vi "GUI_kHz_AlpaoWFS.vi"() -> ()   [LabVIEW 2020]
uses:
  Shared/GUI_Template/GUI_master/tcp_new_data_event.ctl
  Shared/GUI_Template/GUI_master/tcp new data cluster.ctl
  <vilib>/vision/Image Controls.llb/IMAQ Image.ctl
  <vilib>/vision/NI_Vision_Development_Module.lvlib
panel:
  in  "save::1":bool caption="Save"
  in  "exposure::1":dbl=1.005311 caption="Exposure" min=0.001 max=10000.0 format="%_3p"
  in  "cameraselect::1":enum16{"temporal CAM", "spatial CAM"}(ring) caption="Select Camera"
  in  "triggermode::1":bool=TRUE caption="Blank Button"
  in  "Select device":string(combo)="kHz_WFS_Alpao"
  out "tcp data event 2":T1
  out "Tank":dbl(slide)=42.0 scale=0.0..255.0 scale format="%#_6p"
  out "131":T2(plugin-control) caption="Raw Image"
  out "error out":errorcluster
  in  "UDP error message":string
  in  "Refresh Button":bool
  out "GUIdevice 1":string="kHz_AlpaoWFS"
  out "SpatialImage::1":T2(plugin-control) caption="Spatial Image"
  out "frogTrace::1":T2(plugin-control) caption="FROG Trace"
  in  "insert tag":bool=TRUE
  in  "stop":bool
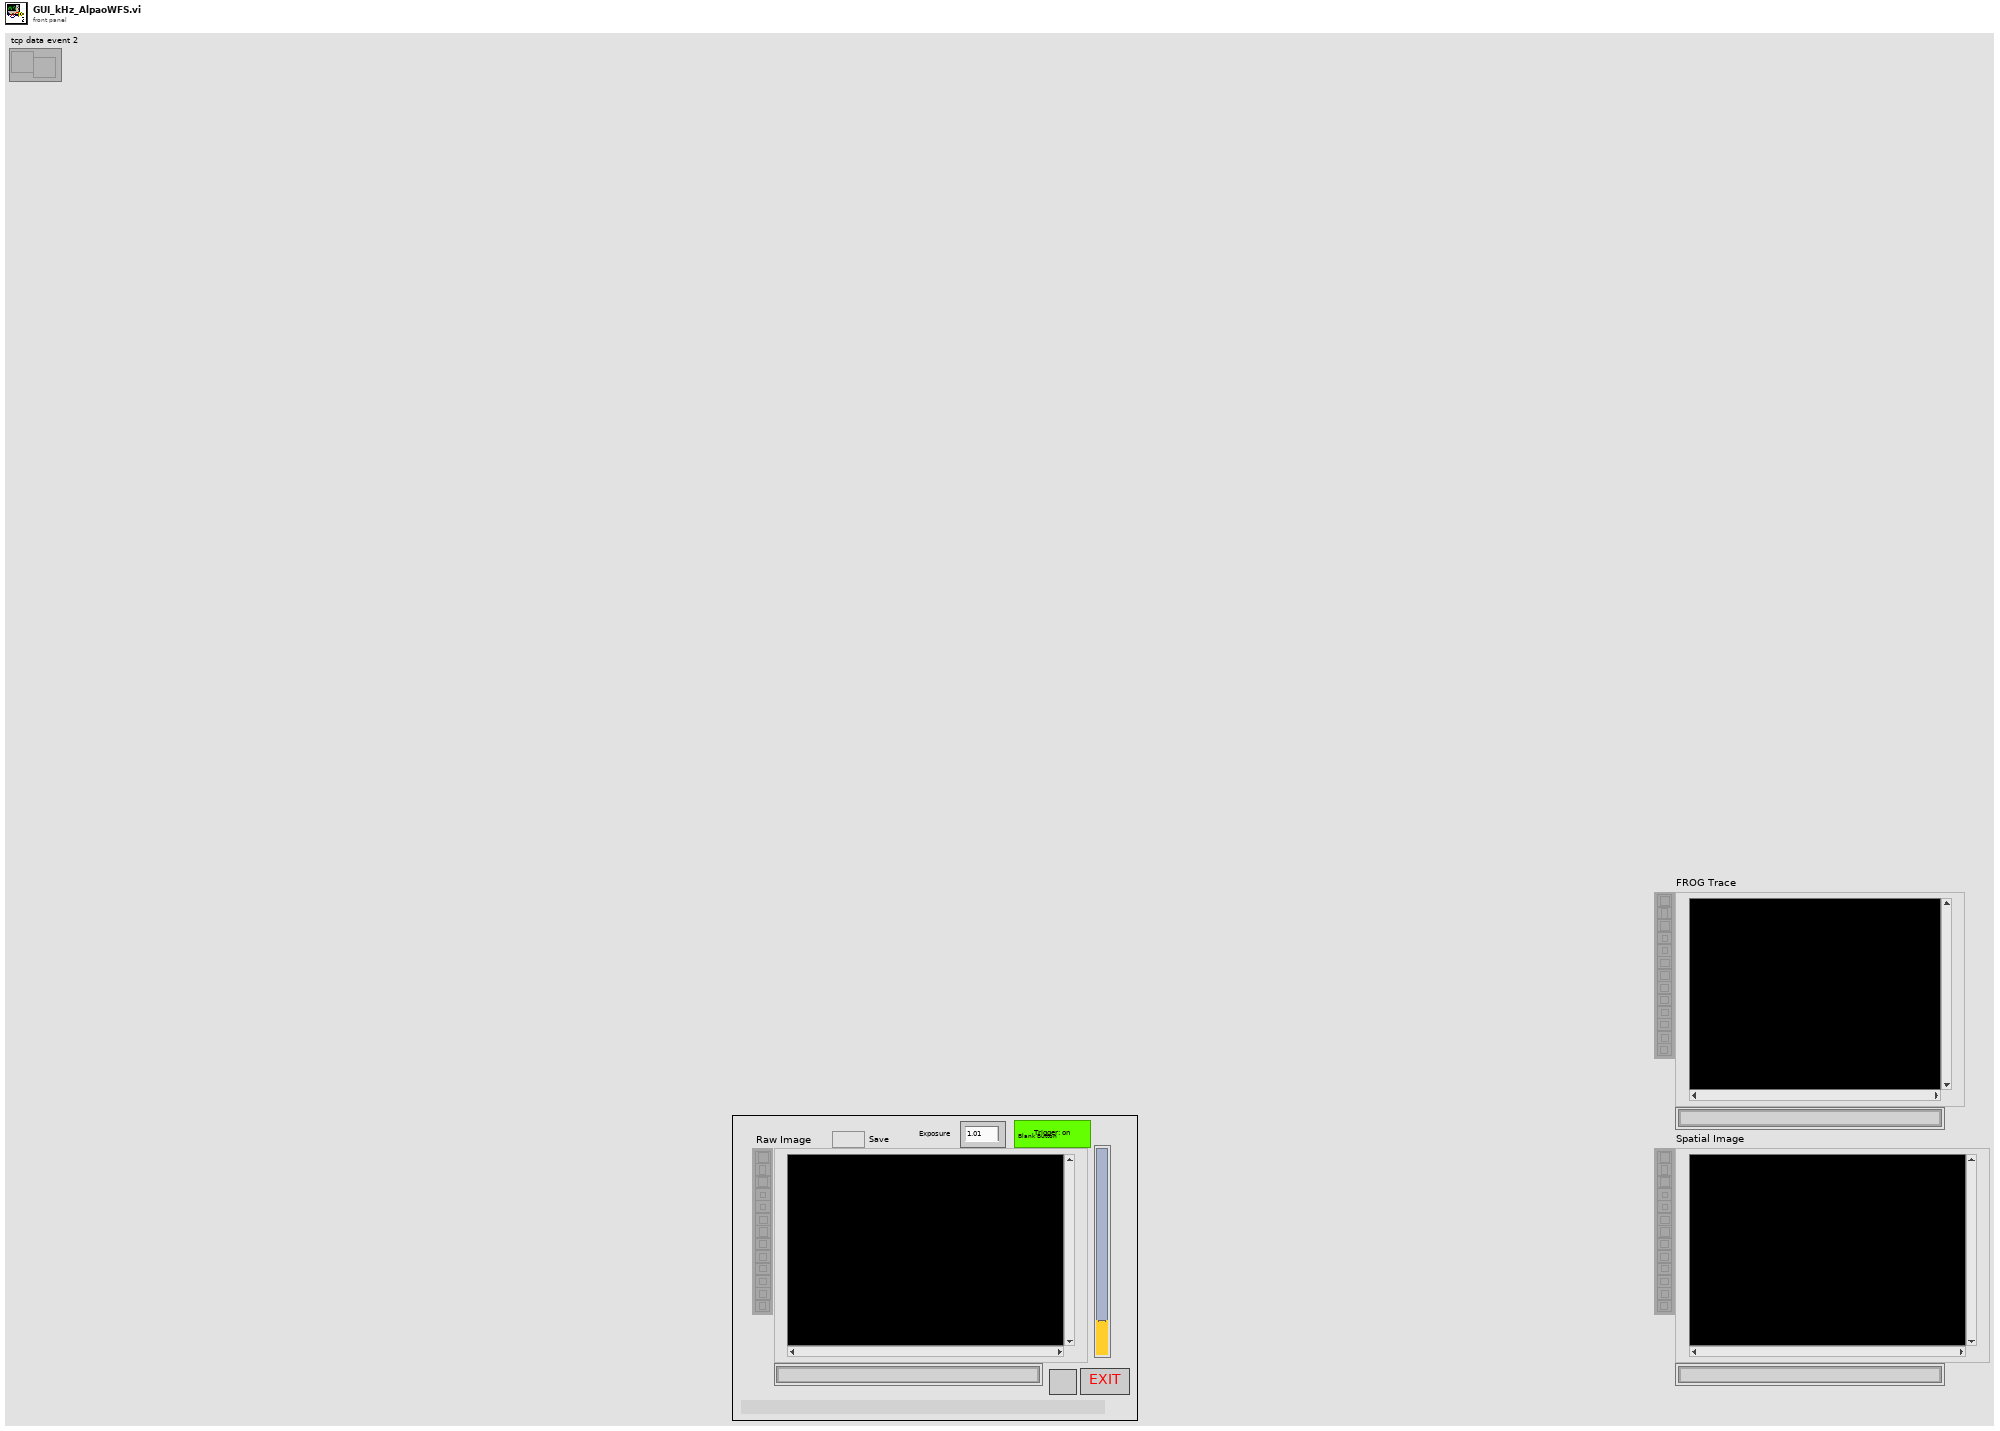
[diagram p1: front panel]
types:
  T1 = typedef "tcp_new_data_event.ctl" = refnum<user-event>
  T2 = typedef "IMAQ Image.ctl" = refnum<image>
  T3 = enum32{"invalid app kind", "Development System", "Run Time System", "Student Edition", "Embedded LabVIEW", "Evaluation", "Custom"}
  T4 = typedef "tcp new data cluster.ctl" = cluster{"EventEnum":enum16{"new data", "connection status update"}, "Device name":string}
  T5 = enum32{"Invalid", "Standard", "Closed", "Hidden", "Minimized", "Maximized"}
  T6 = cluster{"Left":i32, "Top":i32, "Right":i32, "Bottom":i32}
  T7 = cluster{"Core":cluster{"Current VI Reference":refnum<vi>, "Close Panel on Exit?":bool}, "Your Boolean data":bool, "Your string data":string, "SuperGUI":cluster{"STOP queue":refnum<queue>, "SuperGUI ref":refnum<vi>, "event reg":refnum<event-registration>}, "Images":cluster{"frogTrace::1":T2, "retrievedFrogTrace::1":T2, "SpatialImage::1":T2, "rotated_Temporal":T2, "rotated_Spatial":T2}}
  T8 = cluster{"frogTrace::1":T2, "retrievedFrogTrace::1":T2, "SpatialImage::1":T2, "rotated_Temporal":T2, "rotated_Spatial":T2}
  T9 = cluster{"STOP queue":refnum<queue>, "SuperGUI ref":refnum<vi>, "event reg":refnum<event-registration>}
  T10 = cluster{"Current VI Reference":refnum<vi>, "Close Panel on Exit?":bool}
  T11 = typedef "Image Type" = u32
  T12 = cluster{"histogram":u32[], "Minimal Value":sgl, "Maximal Value":sgl, "Starting Value":sgl, "Interval Width":sgl, "Mean Value":sgl, "Standard  Variation":sgl, "Area (pixels)":i32}
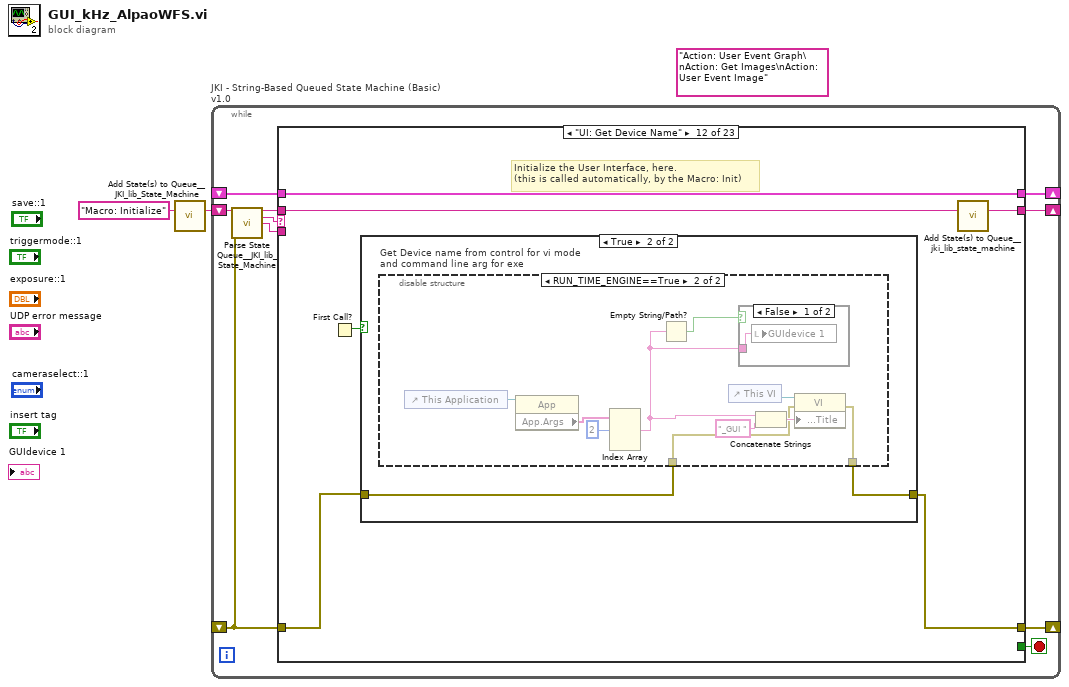
[diagram p0: block diagram]
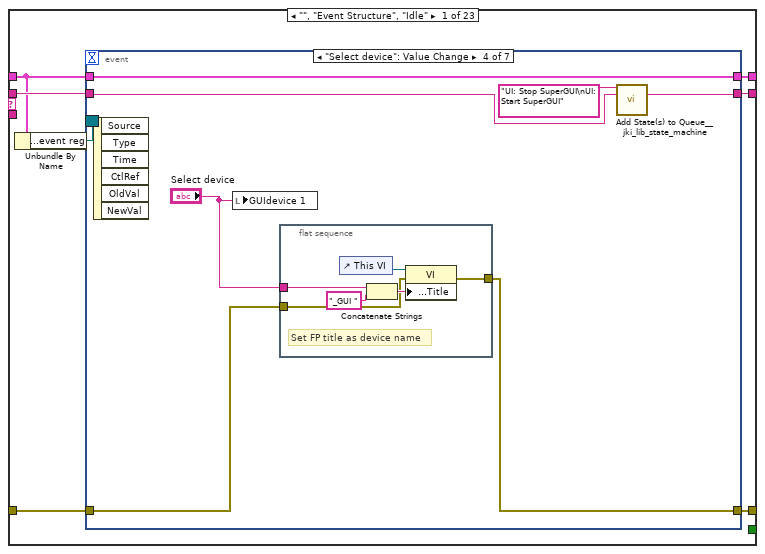
[diagram p2: hidden frame]
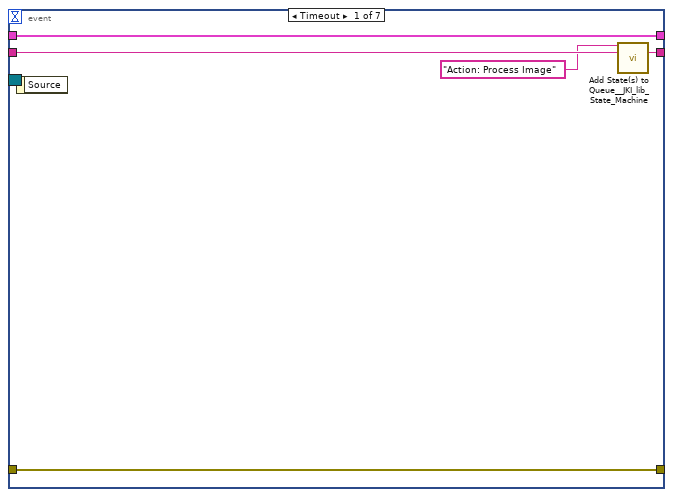
[diagram p3: hidden frame]
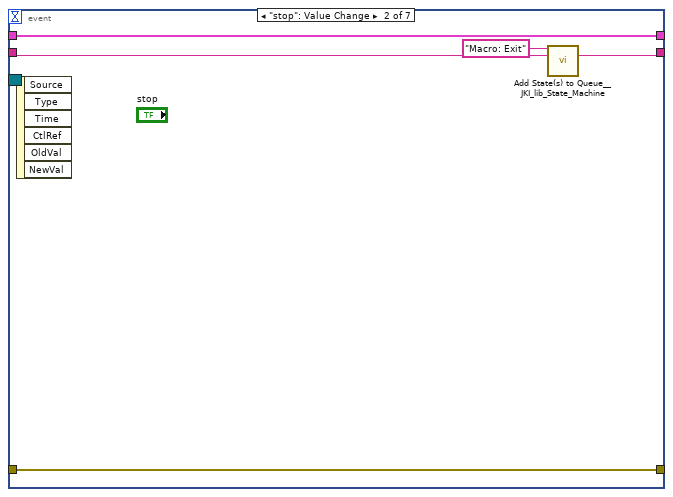
[diagram p4: hidden frame]
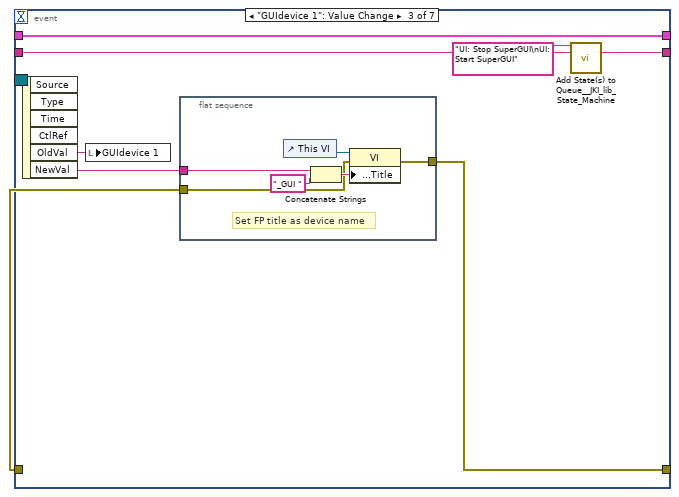
[diagram p5: hidden frame]
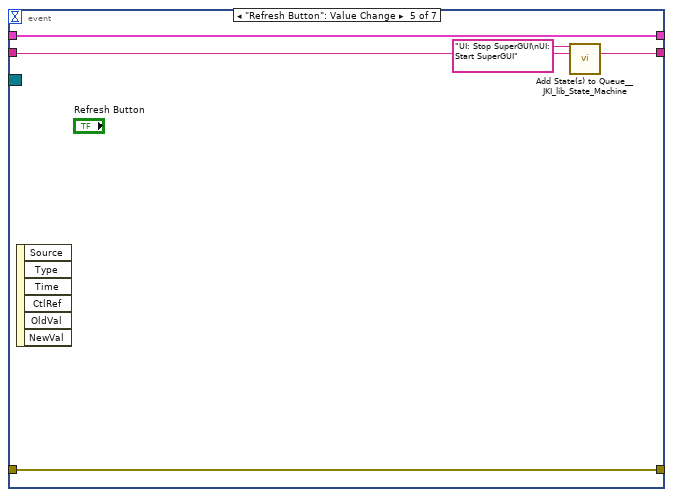
[diagram p6: hidden frame]
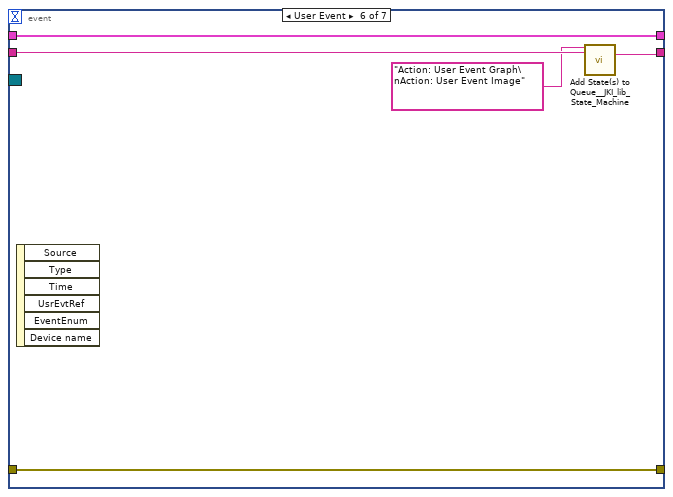
[diagram p7: hidden frame]
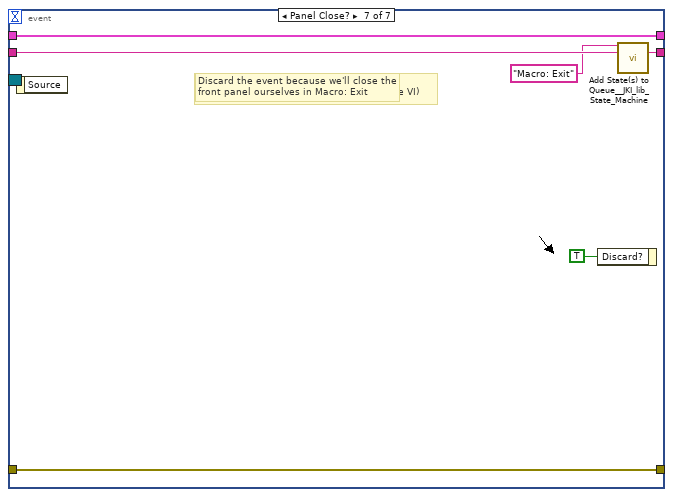
[diagram p8: hidden frame]
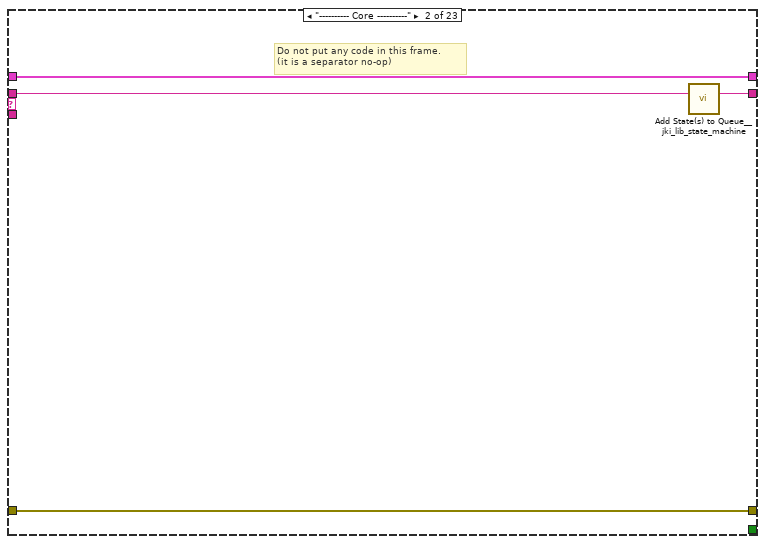
[diagram p9: hidden frame]
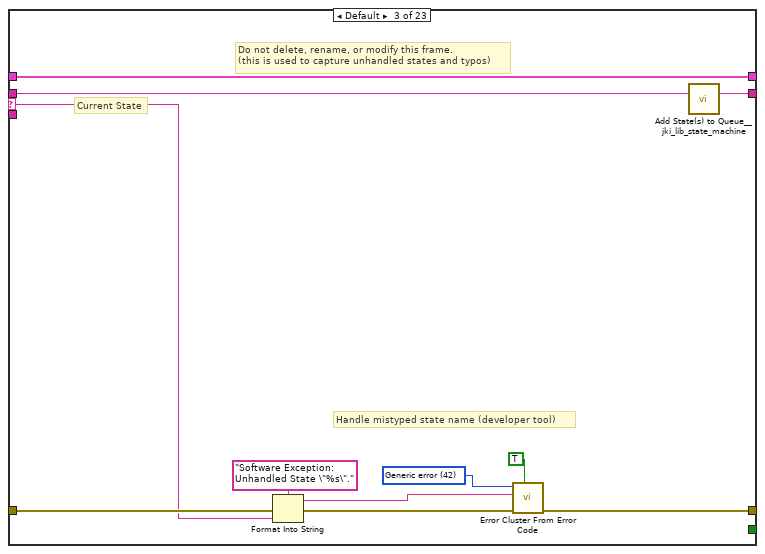
[diagram p10: hidden frame]
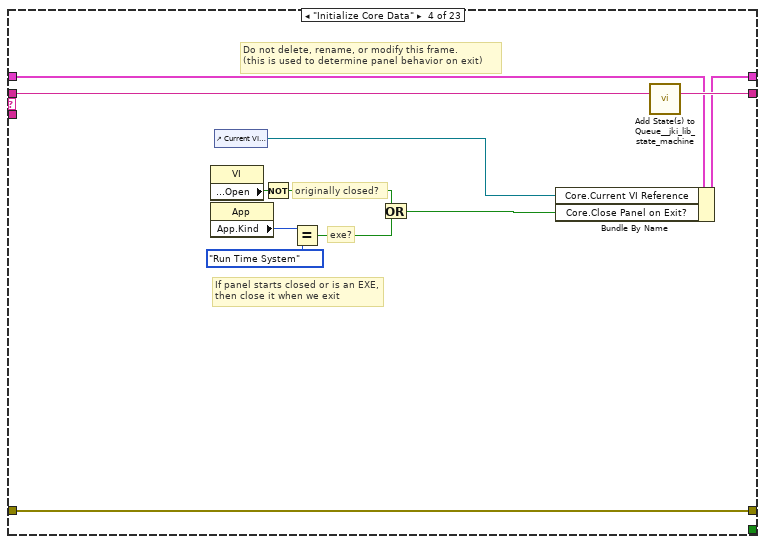
[diagram p11: hidden frame]
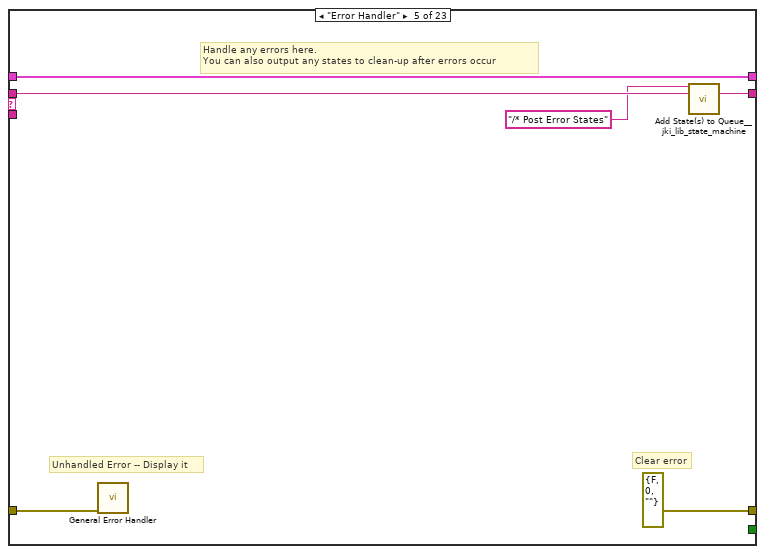
[diagram p12: hidden frame]
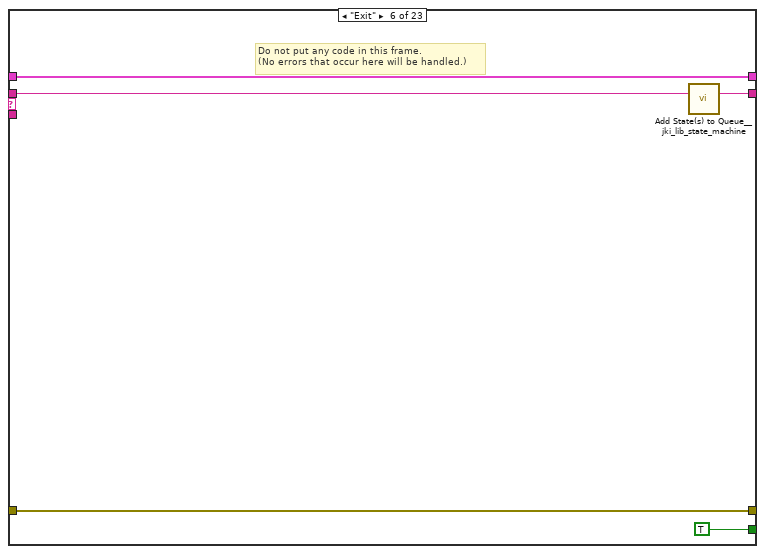
[diagram p13: hidden frame]
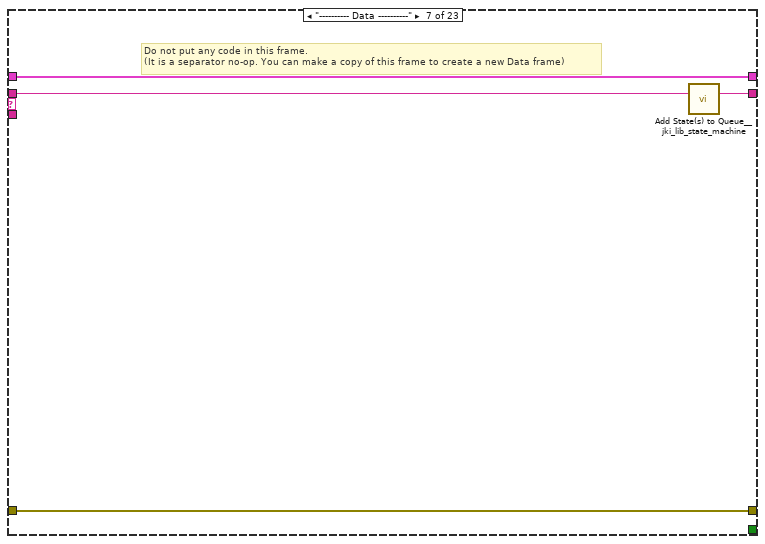
[diagram p14: hidden frame]
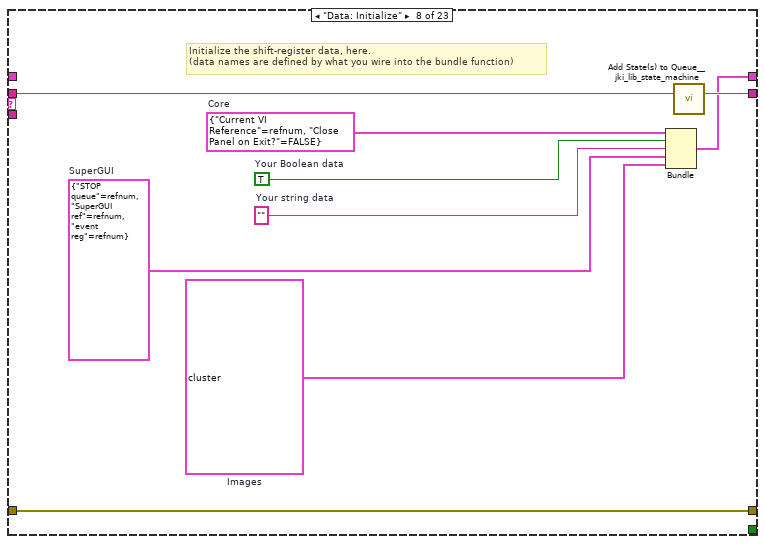
[diagram p15: hidden frame]
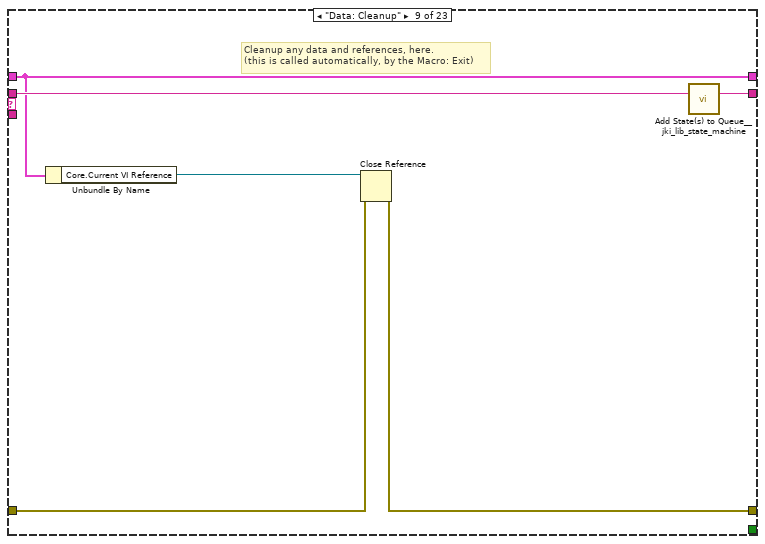
[diagram p16: hidden frame]
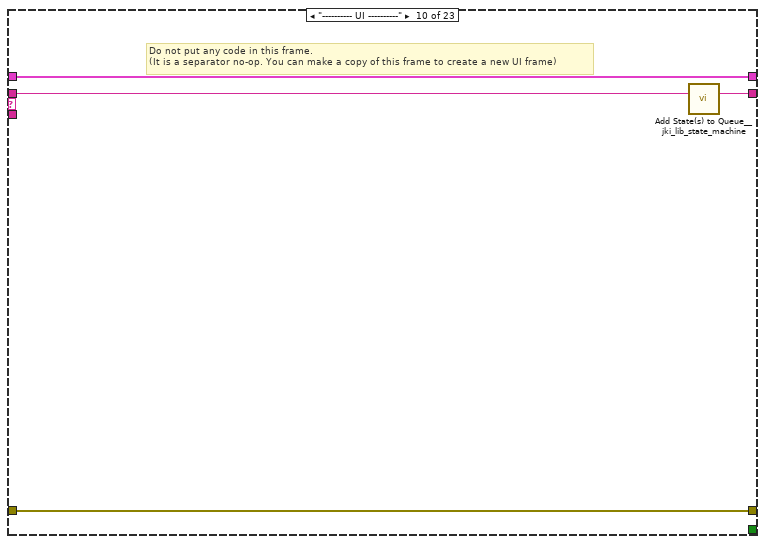
[diagram p17: hidden frame]
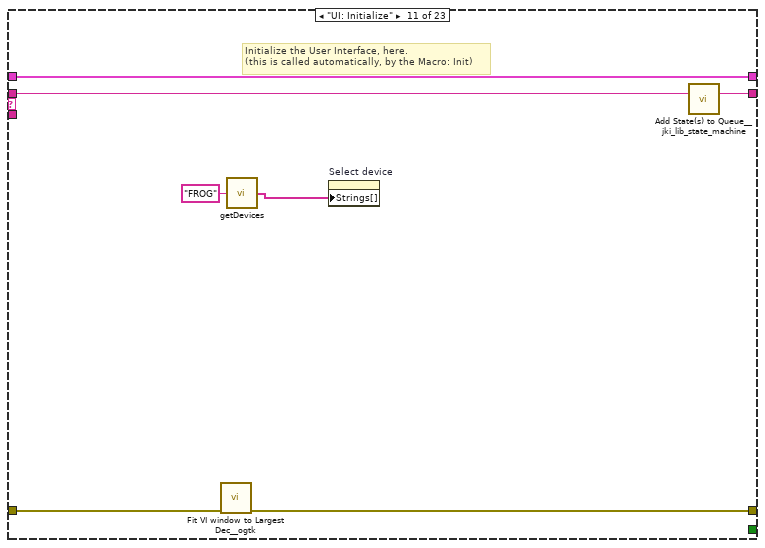
[diagram p18: hidden frame]
diagram:
  (unwired) "Action: User Event Graph\nAction: Get Images\nAction: User Event Image" ("State(s) in Front (\"\")")
  n1 = call <vilib>:"Add State(s) to Queue__JKI_lib_State_Machine.vi"("State(s) in (\"\")"="Macro: Initialize") -> ("States Out"=w2:string)  [unwired: 14 in]
  n2 = while "JKI - String-Based Queued State Machine (Basic) v1.0" {
    shift-right: [w5] -> _
    shift-left: _ -> [w4]
    shift-right: [w8] -> _
    shift-left: _ -> [w3]
    shift-right: [w7] -> _
    shift-left: w2 -> [w9]
    stop <- w6 stop-if-true
    n3 = call <vilib>:"Parse State Queue__JKI_lib_State_Machine.vi"("State Queue"=w9, "Error In (no error)"=w3) -> ("Remaining States"=w11:string, "Current State"=w12:string, "Arguments"=w10:string)  [unwired: 11 in]
    n4 = case shown="\"UI: Get Device Name\"" w12 {
      selector: w12 -> [_ _ w76 _ _ _ _ _ _ _ _ _ _ _ _ _ _ _ _ _ _ _ _]
      tunnel: w11 -> [w19 w75 w80 w98 w104 w109 w113 w122 w128 w132 w139 w145 w182 w190 w196 w207 w233 w238 w248 w252 w256 w276 w291]
      tunnel: w10 -> [_ _ _ _ _ _ _ _ _ _ _ _ _ _ w191 w201 _ _ _ _ _ _ _]
      tunnel: w4 -> [w14 w72 w78 w89 w101 w107 w110 _ w123 w129 w137 w143 w173 w185 w194 w203 w230 w235 w245 w249 w253 w263 w279]
      tunnel: [w17 w73 w82 w95 errorcluster {"status"=FALSE, "code"=0, "source"=""} ("error out") w106 w111 w119 w124 w130 w135 w140 w167 w183 w192 w204 w231 w236 w246 w250 w254 w274 w289] -> w8
      tunnel: w3 -> [w16 w73 w81 w95 w100 w106 w111 w119 w125 w130 w136 w141 w168 w184 w193 w205 w231 w236 w246 w250 w254 w274 w289]
      tunnel: [w18 w74 w79 w97 w103 w108 w112 w121 w127 w131 w138 w144 w181 w189 w195 w206 w232 w237 w247 w251 w255 w275 w290] -> w7
      tunnel: [_ _ _ _ _ TRUE _ _ _ _ _ _ _ _ _ _ _ _ _ _ _ _ _] -> w6
      tunnel: [w15 w72 w78 w96 w101 w107 w110 w120 w123 w129 w137 w143 w172 w185 w194 w203 w230 w235 w245 w249 w253 w262 w279] -> w5
      frame "", "Event Structure", "Idle" {
        n5 = Unbundle By Name(w14) -> ("SuperGUI.event reg"=w13:refnum<event-registration>)
        n6 = event shown="[3] \"Select device\": Value Change" {
          selector: w13 -> [_ _ _ _ _ _ _]
          dyn-events: _ -> [_ _ _ _ _ _ _]
          timeout: _ -> [_ _ _ _ _ _ _]
          tunnel: w19 -> [w24 w27 w33 w45 w58 w64 w71]
          tunnel: [w23 w26 w32 w44 w57 w63 w70] -> w18
          tunnel: w14 -> [w21 w29 w36 w49 w60 w65 w68]
          tunnel: [w22 w28 w34 w47 w59 w61 w69] -> w17
          tunnel: w16 -> [w22 w28 w35 w48 w59 w61 w69]
          tunnel: [w21 w29 w36 w49 w60 w65 w68] -> w15
          event Timeout {
            n7 = event-data() -> ()  [unwired: 1 in, 1 out]
            n8 = call <vilib>:"Add State(s) to Queue__JKI_lib_State_Machine.vi"("State(s) in Front (\"\")"="Action: Process Image" ("State(s) in Front (\"\")"), "State(s) in (\"\")"=w24) -> ("States Out"=w23:string)  [unwired: 13 in]
          }
          event "stop": Value Change {
            n9 = event-data() -> ()  [unwired: 1 in, 6 out]
            n10 = call <vilib>:"Add State(s) to Queue__JKI_lib_State_Machine.vi"("State(s) in Front (\"\")"="Macro: Exit", "State(s) in (\"\")"=w27) -> ("States Out"=w26:string)  [unwired: 13 in]
          }
          event "GUIdevice 1": Value Change {
            n11 = event-data() -> ("NewVal"=w30:string)  [unwired: 1 in, 5 out]
            n12 = local write "GUIdevice 1"(w30) -> ()
            n13 = flat-sequence {
              tunnel: [w39] -> w34
              tunnel: w35 -> [w38]
              tunnel: w30 -> [w37]
              frame #0 {
                # "Set FP title as device name"
                n14 = control-ref of="This VI"() -> (w42:refnum<vi>)
                n15 = Concatenate Strings(w37, "_GUI ") -> (w41:string)
                n16 = property class="VI"(reference=w42, error in=w38, "Front Panel.Title"=w41) -> (error out=w39:errorcluster)  [unwired: 1 out]
              }
            }
            n17 = call <vilib>:"Add State(s) to Queue__JKI_lib_State_Machine.vi"("State(s) in Front (\"\")"="UI: Stop SuperGUI\nUI: Start SuperGUI", "State(s) in (\"\")"=w33) -> ("States Out"=w32:string)  [unwired: 13 in]
          }
          event "Select device": Value Change {
            n18 = event-data() -> ()  [unwired: 1 in, 6 out]
            n19 = local write "GUIdevice 1"("Select device") -> ()
            n20 = flat-sequence {
              tunnel: [w52] -> w47
              tunnel: w48 -> [w51]
              tunnel: "Select device" -> [w50]
              frame #0 {
                # "Set FP title as device name"
                n21 = control-ref of="This VI"() -> (w55:refnum<vi>)
                n22 = Concatenate Strings(w50, "_GUI ") -> (w54:string)
                n23 = property class="VI"(reference=w55, error in=w51, "Front Panel.Title"=w54) -> (error out=w52:errorcluster)  [unwired: 1 out]
              }
            }
            n24 = call <vilib>:"Add State(s) to Queue__jki_lib_state_machine.vi"("State(s) in Front (\"\")"="UI: Stop SuperGUI\nUI: Start SuperGUI", "State(s) in (\"\")"=w45) -> ("States Out"=w44:string)  [unwired: 13 in]
          }
          event "Refresh Button": Value Change {
            n25 = event-data() -> ()  [unwired: 1 in, 6 out]
            n26 = call <vilib>:"Add State(s) to Queue__JKI_lib_State_Machine.vi"("State(s) in Front (\"\")"="UI: Stop SuperGUI\nUI: Start SuperGUI", "State(s) in (\"\")"=w58) -> ("States Out"=w57:string)  [unwired: 13 in]
          }
          event User Event {
            n27 = event-data() -> ()  [unwired: 1 in, 6 out]
            n28 = call <vilib>:"Add State(s) to Queue__JKI_lib_State_Machine.vi"("State(s) in Front (\"\")"="Action: User Event Graph\nAction: User Event Image" ("State(s) in Front (\"\")"), "State(s) in (\"\")"=w64) -> ("States Out"=w63:string)  [unwired: 13 in]
          }
          event Panel Close? {
            # "Discard the event because we'll close the front panel ourselves in Macro: Exit"
            # "Close Panel button (pressed) Event\n(this executes Macro: Exit to terminate the VI)"
            n29 = event-data() -> ()  [unwired: 1 in, 1 out]
            n30 = event-data("Discard?"=TRUE) -> ()  [unwired: 1 in, 1 out]
            n31 = call <vilib>:"Add State(s) to Queue__JKI_lib_State_Machine.vi"("State(s) in Front (\"\")"="Macro: Exit", "State(s) in (\"\")"=w71) -> ("States Out"=w70:string)  [unwired: 13 in]
          }
        }
      }
      frame "---------- Core ----------" {
        # "Do not put any code in this frame.\n(it is a separator no-op)"
        n32 = call <vilib>:"Add State(s) to Queue__jki_lib_state_machine.vi"("State(s) in (\"\")"=w75) -> ("States Out"=w74:string)  [unwired: 14 in]
      }
      frame Default {
        w85 = 42 items=["No error", "Argument error", "Memory is full", "Out of zone", "End of file", "File already open", "Generic file I/O error", "File not found", "File permission error", "Disk is full", "Duplicate path", "Too many files open", "System feature not enabled", "Resource file not found", "Cannot add resource", "Resource not found", "Image not found", "Image memory error", "Pen does not exist", "Config type invalid", "Config token not found", "Config parse error", "Config memory error", "Bad external code format", "Bad external code offset", "External code not present", "Null window", "Destroy window error", "Null menu", "Print aborted", "Bad print record", "Print driver error", "Windows error during printing", "Memory error during printing", "Print dialog error", "Generic print error", "Invalid device refnum", "Device not found", "Device parameter error", "Device unit error", "Cannot open device", "Device call aborted", "Generic error", "Cancelled by user", "Object ID too low", "Object ID too high", "Object not in heap", "Unknown heap", "Unknown object (invalid DefProc)", "Unknown object (DefProc not in table)", "Message out of range", "Invalid (null) method", "Unknown message", "Manager call not supported", "Bad address", "Network operation in progress", "Network operation timed out", "Connection is busy", "Network attribute not supported", "Network error", "Address in use", "System out of memory", "Connection aborted", "Connection refused", "Not connected", "Already connected", "Connection closed", "Initialization error (interapplication manager)", "Bad occurrence", "Wait on unbound occurrence handler", "Occurrence queue overflow", "Datalog type conflict", "Unused", "Unrecognized type (interapplication manager)", "Memory corrupt", "Failed to make temporary DLL", "Old CIN version", "Drag socket not found", "Failed to load drop-object", "Failed to register OLE object", "Failed to release OLE object", "Format specifier type mismatch", "Unknown format specifier", "Too few format specifiers", "Too many format specifiers", "Scan failed", "Newer CIN version", "Error converting to variant", "Runtime menu error", "Password tampered", "Variant attribute not found", "Incompatible variant data type", "Event data is not available", "Event Store is not present", "Occurrence is not found", "Event Queue is not created", "Event info is not available", "Refnum passed is NULL", "Error retrieving Class GUID", "Error retrieving CoClass GUID", "Error retrieving TypeLib GUID.", "Bad built application magic bytes.", "Specific driver is different from the specific driver associated with the Logical Name.", "There is no session opened to the class driver.", "Max Error", "MAX - Error with config objects", "MAX - Error loading configuration", "MAX - Group not supported"]
        # "Current State"
        # "Do not delete, rename, or modify this frame.\n(this is used to capture unhandled states and typos)"
        # "Handle mistyped state name (developer tool)"
        n33 = Format Into String(format string="Software Exception: Unhandled State \"%s\"." ("message"), error in=w81, w76) -> (resulting string=w84:string, error out=w83:errorcluster)  [unwired: 1 in]
        n34 = call <vilib>:"Error Cluster From Error Code.vi"("show call chain? (False)"=TRUE, "error in (no error)"=w83, "error message (\"\")"=w84, "error code (0)"=w85) -> ("error out"=w82:errorcluster)  [unwired: 5 in]
        n35 = call <vilib>:"Add State(s) to Queue__jki_lib_state_machine.vi"("State(s) in (\"\")"=w80) -> ("States Out"=w79:string)  [unwired: 14 in]
      }
      frame "Initialize Core Data" {
        # "Do not delete, rename, or modify this frame.\n(this is used to determine panel behavior on exit)"
        # "originally closed?"
        # "exe?"
        # "If panel starts closed or is an EXE, then close it when we exit"
        n36 = property class="VI"() -> ("Front Panel.Open"=w94:bool)  [unwired: 2 in, 2 out]
        n37 = property class="App"() -> ("App.Kind"=w93:T3)  [unwired: 2 in, 2 out]
        n38 = control-ref of="Current VI Reference"() -> (w87:refnum<vi>)
        n39 = Not(x=w94) -> (.not. x?=w91:bool)
        n40 = Equal?(x=w93, y=T3."Run Time System" ("Application:Kind")) -> (x = y?=w90:bool)
        n41 = Or(x=w91, y=w90) -> (x .or. y?=w88:bool)
        n42 = Bundle By Name(cluster=w89, "Core.Current VI Reference"=w87, "Core.Close Panel on Exit?"=w88) -> (w96:T7)
        n43 = call <vilib>:"Add State(s) to Queue__jki_lib_state_machine.vi"("State(s) in (\"\")"=w98) -> ("States Out"=w97:string)  [unwired: 14 in]
      }
      frame "Error Handler" {
        # "Unhandled Error -- Display it"
        # "Handle any errors here.\nYou can also output any states to clean-up after errors occur"
        # "Clear error"
        n44 = call <vilib>:"General Error Handler.vi"("error in (no error)"=w100) -> ()  [unwired: 10 in, 5 out]
        n45 = call <vilib>:"Add State(s) to Queue__jki_lib_state_machine.vi"("State(s) in Front (\"\")"="/* Post Error States", "State(s) in (\"\")"=w104) -> ("States Out"=w103:string)  [unwired: 13 in]
      }
      frame "Exit" {
        # "Do not put any code in this frame.\n(No errors that occur here will be handled.)"
        n46 = call <vilib>:"Add State(s) to Queue__jki_lib_state_machine.vi"("State(s) in (\"\")"=w109) -> ("States Out"=w108:string)  [unwired: 14 in]
      }
      frame "---------- Data ----------" {
        # "Do not put any code in this frame.\n(It is a separator no-op. You can make a copy of this frame to create a new Data frame)"
        n47 = call <vilib>:"Add State(s) to Queue__jki_lib_state_machine.vi"("State(s) in (\"\")"=w113) -> ("States Out"=w112:string)  [unwired: 14 in]
      }
      frame "Data: Initialize" {
        w114 = T8 {"frogTrace::1"="remote image 000000001E51927C", "retrievedFrogTrace::1"="remote image 000000001E51927C", "SpatialImage::1"="remote image 000000001E51927C", "rotated_Temporal"=refnum, "rotated_Spatial"=refnum}  # Images
        w115 = T9 {"STOP queue"=refnum, "SuperGUI ref"=refnum, "event reg"=refnum}  # SuperGUI
        w116 = T10 {"Current VI Reference"=refnum, "Close Panel on Exit?"=FALSE}  # Core
        w118 = TRUE  # Your Boolean data
        w117 = ""  # Your string data
        # "Initialize the shift-register data, here.\n(data names are defined by what you wire into the bundle function)"
        n48 = Bundle("Core"=w116, "Your Boolean data"=w118, "Your string data"=w117, "SuperGUI"=w115, "Images"=w114) -> (w120:T7)  [unwired: 1 in]
        n49 = call <vilib>:"Add State(s) to Queue__jki_lib_state_machine.vi"("State(s) in (\"\")"=w122) -> ("States Out"=w121:string)  [unwired: 14 in]
      }
      frame "Data: Cleanup" {
        # "Cleanup any data and references, here.\n(this is called automatically, by the Macro: Exit)"
        n50 = Unbundle By Name(w123) -> ("Core.Current VI Reference"=w126:refnum<vi>)
        n51 = Close Reference(reference=w126, error in (no error)=w125) -> (error out=w124:errorcluster)
        n52 = call <vilib>:"Add State(s) to Queue__jki_lib_state_machine.vi"("State(s) in (\"\")"=w128) -> ("States Out"=w127:string)  [unwired: 14 in]
      }
      frame "---------- UI ----------" {
        # "Do not put any code in this frame.\n(It is a separator no-op. You can make a copy of this frame to create a new UI frame)"
        n53 = call <vilib>:"Add State(s) to Queue__jki_lib_state_machine.vi"("State(s) in (\"\")"=w132) -> ("States Out"=w131:string)  [unwired: 14 in]
      }
      frame "UI: Initialize" {
        # "Initialize the User Interface, here.\n(this is called automatically, by the Macro: Init)"
        n54 = call <userlib>:"Fit VI window to Largest Dec__ogtk.vi"("error in (no error)"=w136) -> ("error out"=w135:errorcluster)  [unwired: 5 in, 1 out]
        n55 = call "getDevices.vi"("Device Class"="FROG") -> ("All Devices"=w133:string[])
        n56 = property on="Select device" class="CmbBox"("Strings[]"=w133) -> ()  [unwired: 2 in, 2 out]
        n57 = call <vilib>:"Add State(s) to Queue__jki_lib_state_machine.vi"("State(s) in (\"\")"=w139) -> ("States Out"=w138:string)  [unwired: 14 in]
      }
      frame "UI: Get Device Name" {
        # "Initialize the User Interface, here.\n(this is called automatically, by the Macro: Init)"
        n58 = First Call?() -> (First Call?: T/F=w142:bool)
        n59 = case shown="True" w142 {
          tunnel: w141 -> [w146 w148]
          tunnel: [w146 w147] -> w140
          frame False {
          }
          frame True {
            n60 = disable-structure "Get Device name from control for vi mode\nand command line arg for exe" shown="RUN_TIME_ENGINE==True" {
              disable-tunnel: w148 -> [w149 w151]
              disable-tunnel: [w149 w150] -> w147
              frame condition #0 (active) {
              }
              frame condition #1 {
                n61 = control-ref of="This Application"() -> (w159:refnum<vi>)
                n62 = property class="App"(reference=w159) -> ("App.Args"=w158:string[])  [unwired: 1 in, 2 out]
                n63 = Index Array(array=w158, index #1=2 ("index")) -> (element #1=w152:string)  [unwired: 2 in, 2 out]
                n64 = Empty String/Path?(string/path=w152) -> (empty?=w156:bool)
                n65 = control-ref of="This VI"() -> (w155:refnum<vi>)
                n66 = case shown="False" w156 {
                  tunnel: w152 -> [w160 _]
                  frame False {
                    n67 = local write "GUIdevice 1"(w160) -> ()
                  }
                  frame True {
                  }
                }
                n68 = Concatenate Strings(w152, "_GUI ") -> (w154:string)
                n69 = property class="VI"(reference=w155, error in=w151, "Front Panel.Title"=w154) -> (error out=w150:errorcluster)  [unwired: 1 out]
              }
            }
          }
        }
        n70 = call <vilib>:"Add State(s) to Queue__jki_lib_state_machine.vi"("State(s) in (\"\")"=w145) -> ("States Out"=w144:string)  [unwired: 14 in]
      }
      frame "UI: Start SuperGUI" {
        # "create stop queue for supergui and its clones"
        # "x100 abort will be dependent on caller VI\nx80 abort will be independent of caller vi, this will abort vi when labview is closed."
        # "Start SuperGUI asynchronous way"
        n71 = vi-ref "GUI_Master_subvi_reentrant_queues.vi"() -> (w166:refnum<vi>)
        n72 = property class="VI"(reference=w166) -> ("Path"=w165:path)  [unwired: 1 in, 2 out]
        n73 = Create User Event(user event datatype=T4 {"EventEnum"=enum."new data", "Device name"="Device name"} ("New Event"), error in=w168) -> (user event=w163:refnum<user-event>, error out=w174:errorcluster)
        "tcp data event 2" <- w163
        n74 = control-ref of="This Application"() -> (w171:refnum<vi>)
        n75 = control-ref of="This VI"() -> (w170:refnum<vi>)
        n76 = Open VI Reference(type specifier VI Refnum (for type only)=refnum<vi> refnum, vi path=w165, options=256) -> (vi reference=w180:refnum<vi>, error out=w179:errorcluster)  [unwired: 3 in]
        n77 = register-events(w163) -> (reference out=w162:refnum<event-registration>)  [unwired: 2 in, 1 out]
        n78 = call "supergui create stop queue.vi"() -> ("STOP Queue out"=w176:refnum<queue>)  [unwired: 11 in]
        n79 = Current VI's Menubar() -> (w169:refnum<k9>)
        n80 = call-by-ref "Start Asynchronous Call"(reference=w180, error in=w179, "STOP Queue in"=w176, "This Application"=w171, 8:"error in (no error)"=w174, "tcp data event"=w163, "Caller menu reference"=w169, "Caller VI ref"=w170) -> (reference out=w164:refnum<vi>, error out=w167:errorcluster)  [unwired: 5 in, 1 out]
        n81 = Bundle By Name(cluster=w173, "SuperGUI.event reg"=w162, "SuperGUI.SuperGUI ref"=w164, "SuperGUI.STOP queue"=w176) -> (w172:T7)
        n82 = call <vilib>:"Add State(s) to Queue__jki_lib_state_machine.vi"("State(s) in Front (\"\")"="Action: Get Images" ("State(s) in Front (\"\")"), "State(s) in (\"\")"=w182) -> ("States Out"=w181:string)  [unwired: 13 in]
      }
      frame "UI: Stop SuperGUI" {
        # "Stop Supergui Clone and wait until it exit properly"
        n83 = Unbundle By Name(w185) -> ("SuperGUI.SuperGUI ref"=w187:refnum<vi>, "SuperGUI.STOP queue"=w186:refnum<queue>)
        n84 = Release Queue(queue=w186, error in (no error)=w184) -> (error out=w188:errorcluster)  [unwired: 1 in, 2 out]
        n85 = call-by-ref "Wait On Asynchronous Call"(reference=w187, error in=w188) -> ("error out"=w183:errorcluster)  [unwired: 11 in, 2 out]
        n86 = call <vilib>:"Add State(s) to Queue__jki_lib_state_machine.vi"("State(s) in (\"\")"=w190) -> ("States Out"=w189:string)  [unwired: 14 in]
      }
      frame "UI: Cursor Set" {
        # "Argument"
        # "Set and Unset Cursor Busy.\n(Usage: \"UI: Cursor Set >> Busy|Idle\")"
        n87 = case shown="\"Idle\", Default" w191 {
          tunnel: w193 -> [w198 w200]
          tunnel: [w197 w199] -> w192
          frame "Idle", Default {
            n88 = call <vilib>:"Unset Busy.vi"("error in (no error)"=w198) -> ("error out"=w197:errorcluster)  [unwired: 10 in]
          }
          frame "Busy" {
            n89 = call <vilib>:"Set Busy.vi"("error in (no error)"=w200) -> ("error out"=w199:errorcluster)  [unwired: 9 in, 1 out]
          }
        }
        n90 = call <vilib>:"Add State(s) to Queue__jki_lib_state_machine.vi"("State(s) in (\"\")"=w196) -> ("States Out"=w195:string)  [unwired: 14 in]
      }
      frame "UI: Front Panel State" {
        # "Argument"
        # "Set Front Panel Open or Closed\n(Usage: \"UI: Front Panel State >> Open|Close\")"
        n91 = Unbundle By Name(w203) -> ("Core.Current VI Reference"=w202:refnum<vi>)
        n92 = case shown="\"Open\", Default" w201 {
          tunnel: w205 -> [w211 w224]
          tunnel: [w213 w225] -> w204
          tunnel: w202 -> [w212 w222]
          frame "Open", Default {
            n93 = property class="VI"(reference=w212, error in=w211) -> (reference out=w209:refnum<vi>, error out=w210:errorcluster, "Front Panel.Open"=w208:bool)
            n94 = case shown="False" w208 {
              tunnel: [w216 w219] -> w213
              tunnel: w210 -> [w215 w219]
              tunnel: w209 -> [w214 _]
              frame False {
                n95 = invoke class="VI" method="FP.Open"(reference=w214, error in=w215, "Activate"=TRUE, "State"=T5."Standard") -> (error out=w216:errorcluster)  [unwired: 1 in, 4 out]
              }
              frame True {
              }
            }
          }
          frame "Close" {
            n96 = property class="VI"(reference=w222, error in=w224) -> (reference out=w221:refnum<vi>, error out=w223:errorcluster, "Front Panel.Open"=w220:bool)
            n97 = case shown="True" w220 {
              tunnel: [w226 w229] -> w225
              tunnel: w223 -> [w226 w228]
              tunnel: w221 -> [_ w227]
              frame False {
              }
              frame True {
                n98 = invoke class="VI" method="FP.Close"(reference=w227, error in=w228) -> (error out=w229:errorcluster)  [unwired: 1 in, 2 out]
              }
            }
          }
        }
        n99 = call <vilib>:"Add State(s) to Queue__jki_lib_state_machine.vi"("State(s) in (\"\")"=w207) -> ("States Out"=w206:string)  [unwired: 14 in]
      }
      frame "---------- Macro ----------" {
        # "Do not put any code in this frame.\n(It is a separator no-op. You can make a copy of this frame to create a new Macro frame)"
        n100 = call <vilib>:"Add State(s) to Queue__jki_lib_state_machine.vi"("State(s) in (\"\")"=w233) -> ("States Out"=w232:string)  [unwired: 14 in]
      }
      frame "Macro: Initialize" {
        # "Initialization Macro\n(This is called once, when the VI starts)"
        n101 = call <vilib>:"Add State(s) to Queue__jki_lib_state_machine.vi"("State(s) in Front (\"\")"="Data: Initialize\nInitialize Core Data\nUI: Initialize\nUI: Get Device Name\nUI: Start SuperGUI\nUI: Front Panel State >> Open", "State(s) in (\"\")"=w238) -> ("States Out"=w237:string)  [unwired: 13 in]
      }
      frame "Macro: Exit" {
        # "Exit Macro\n(This is called once, when the VI exits)"
        n102 = Unbundle By Name(w245) -> ("Core.Close Panel on Exit?"=w244:bool)
        n103 = Select(t="UI: Front Panel State >> Close", s=w244, f="") -> (s? t:f=w241:string)
        n104 = call <vilib>:"Add State(s) to Queue__jki_lib_state_machine.vi"("State(s) in (\"\")"=w241, "State(s) at Back (\"\")"="Data: Cleanup\nExit") -> ("States Out"=w239:string)  [unwired: 13 in]
        n105 = call <vilib>:"Add State(s) to Queue__jki_lib_state_machine.vi"("State(s) in Front (\"\")"=w239, "State(s) in (\"\")"=w248) -> ("States Out"=w247:string)  [unwired: 13 in]
      }
      frame "---------- New Category ----------" {
        # "Template Separator\n(You can make a copy of, or modify, this frame)"
        n106 = call <vilib>:"Add State(s) to Queue__jki_lib_state_machine.vi"("State(s) in (\"\")"=w252) -> ("States Out"=w251:string)  [unwired: 14 in]
      }
      frame "Action: User Event Graph" {
        n107 = call <vilib>:"Add State(s) to Queue__jki_lib_state_machine.vi"("State(s) in (\"\")"=w256) -> ("States Out"=w255:string)  [unwired: 14 in]
      }
      frame "Action: Get Images" {
        w270 = T11 0 items=["Grayscale (U8)", "Grayscale (I16)", "Grayscale (SGL)", "Complex (CSG)", "RGB (U32)", "HSL (U32)", "RGB (U64)", "Grayscale (U16)"] ("Image Type")
        w273 = T11 0 items=["Grayscale (U8)", "Grayscale (I16)", "Grayscale (SGL)", "Complex (CSG)", "RGB (U32)", "HSL (U32)", "RGB (U64)", "Grayscale (U16)"] ("Image Type")
        w264 = T11 0 items=["Grayscale (U8)", "Grayscale (I16)", "Grayscale (SGL)", "Complex (CSG)", "RGB (U32)", "HSL (U32)", "RGB (U64)", "Grayscale (U16)"] ("Image Type")
        w267 = T11 0 items=["Grayscale (U8)", "Grayscale (I16)", "Grayscale (SGL)", "Complex (CSG)", "RGB (U32)", "HSL (U32)", "RGB (U64)", "Grayscale (U16)"] ("Image Type")
        w268 = T11 0 items=["Grayscale (U8)", "Grayscale (I16)", "Grayscale (SGL)", "Complex (CSG)", "RGB (U32)", "HSL (U32)", "RGB (U64)", "Grayscale (U16)"] ("Image Type")
        n108 = call "IMAQ Create"("Image Name"="retrievedFrogTrace::1", "Image Type"=w267) -> ("New Image"=w260:T2)  [unwired: 3 in, 1 out]
        n109 = call "IMAQ Create"("Image Name"="frogTrace::1", "Image Type"=w268) -> ("New Image"=w261:T2)  [unwired: 3 in, 1 out]
        "frogTrace::1" <- w261
        n110 = call "IMAQ Create"("Image Name"="SpatialImage::1", "Image Type"=w264) -> ("New Image"=w259:T2)  [unwired: 3 in, 1 out]
        "SpatialImage::1" <- w259
        n111 = call "IMAQ Create"("Image Name"="rotated_Spatial", "Image Type"=w270) -> ("New Image"=w257:T2)  [unwired: 3 in, 1 out]
        n112 = call "IMAQ Create"("Image Name"="rotated_Temporal", "Image Type"=w273) -> ("New Image"=w258:T2)  [unwired: 3 in, 1 out]
        n113 = Bundle By Name(cluster=w263, "Images.frogTrace::1"=w261, "Images.retrievedFrogTrace::1"=w260, "Images.SpatialImage::1"=w259, "Images.rotated_Temporal"=w258, "Images.rotated_Spatial"=w257) -> (w262:T7)
        n114 = call <vilib>:"Add State(s) to Queue__jki_lib_state_machine.vi"("State(s) in (\"\")"=w276) -> ("States Out"=w275:string)  [unwired: 14 in]
      }
      frame "Action: User Event Image" {
        n115 = Unbundle By Name(w279) -> ("Images.frogTrace::1"=w278:T2, "Images.rotated_Temporal"=w277:T2)  [unwired: 2 out]
        n116 = call "IMAQ Rotate"("Maintain Size"=TRUE, "Angle (degrees)"=sgl 0.0, "Image Dst"=w277, "Image Src"=w278) -> ("error out"=w281:errorcluster, "Image Dst Out"=w284:T2)  [unwired: 6 in]
        n117 = call "IMAQ Histogram"("Image"=w278) -> ("Histogram Report"=w287:T12)  [unwired: 9 in, 1 out]
        n118 = call <vilib>:"Clear Errors.vi"("error in (no error)"=w281) -> ("error out"=w285:errorcluster)  [unwired: 5 in, 1 out]
        n119 = disable-structure shown="Enabled" {
          disable-tunnel: [w296 w297] -> w286
          disable-tunnel: w285 -> [w295 w298]
          disable-tunnel: w284 -> [w294 w297]
          disable-tunnel: [w292 w298] -> w283
          frame Disabled {
            (unwired) 384.0 ("Target.Y")
            (unwired) 288.0 ("Target.X")
            (unwired) cluster{"xhair size":dbl, "xhair size 2":dbl} {"xhair size"=275.0, "xhair size 2"=275.0} ("size")
            (unwired) u32 16774656 ("Color")
            n120 = call "draw crosshair imaq.vi"("error in (no error)"=w295, "Bounding Rectangle"=T6 {"Left"=0, "Top"=0, "Right"=0, "Bottom"=0}, "image in"=w294) -> ("error out"=w292:errorcluster, "image out"=w296:T2)  [unwired: 7 in]
          }
          frame Enabled {
          }
        }
        "131" <- w286
        "error out" <- w283
        n121 = Unbundle By Name(w287) -> ("Maximal Value"=→"Tank":sgl)
        n122 = call <vilib>:"Add State(s) to Queue__jki_lib_state_machine.vi"("State(s) in (\"\")"=w291) -> ("States Out"=w290:string)  [unwired: 14 in]
      }
    }
  }
